vi "XML_time.vi"(1 "IP Address of NIST Time Server":string(combo), 2 "NIST Time":u64, 3 "Input String":string) -> (0 "Output String":string)   [LabVIEW 2012]
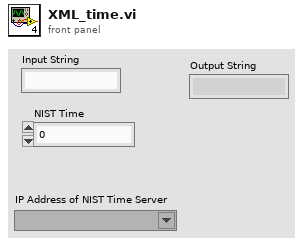
[diagram p1: front panel]
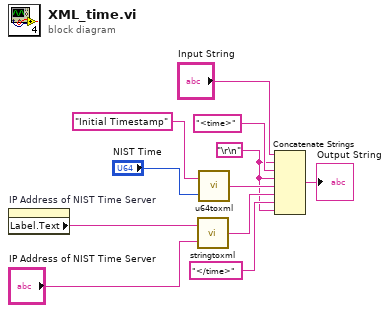
[diagram p0: block diagram]
diagram:
  w5 = "\r\n"
  n1 = property on="IP Address of NIST Time Server" class="CmbBox"() -> ("Label.Text"=w2:string)  [unwired: 2 in, 2 out]
  n2 = call "stringtoxml.vi"("String to write"="IP Address of NIST Time Server", "XML Tag"=w2) -> ("xml string"=w7:string)
  n3 = call "u64toxml.vi"("variable"="NIST Time", "variable name"="Initial Timestamp") -> ("xml string"=w11:string)
  n4 = Concatenate Strings("Input String", w5, "<time>" ("string"), w5, w11, w7, "</time>" ("string"), w5) -> (→"Output String":string)
